vi "BGK8001 Command.vi"(9 "cmd parameter":string caption="指令参数", 10 "cmd code":string caption="指令代码", 11 "unit adress":string caption="设备地址") -> (3 "cmd":string caption="指令")   [LabVIEW 2015]
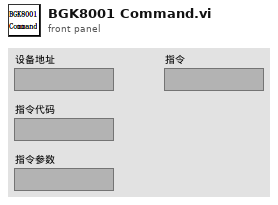
[diagram p1: front panel]
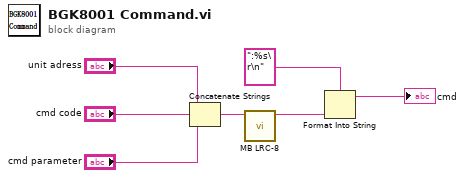
[diagram p0: block diagram]
diagram:
  n1 = Concatenate Strings("unit adress", "cmd code", "cmd parameter") -> (w6:string)
  n2 = call "MB LRC-8.vi"("String"=w6) -> ("string & LRC-8"=w3:string)  [unwired: 8 in, 2 out]
  n3 = Format Into String(format string=":%s\r\n" ("格式字符串"), w3) -> (resulting string=→"cmd":string)  [unwired: 2 in, 1 out]
